vi "Read picture.vi"(8 "error in (no error)":errorcluster, 11 "data_loader in":refnum<class "data_loader.lvclass">) -> (0 "error out":errorcluster, 2 "picture":picture, 3 "data_loader out":refnum<class "data_loader.lvclass">)   [LabVIEW 2017, in "data_loader.lvclass"]
uses:
  data_loader.lvclass
  data_loader.lvclass/data_loader.ctl
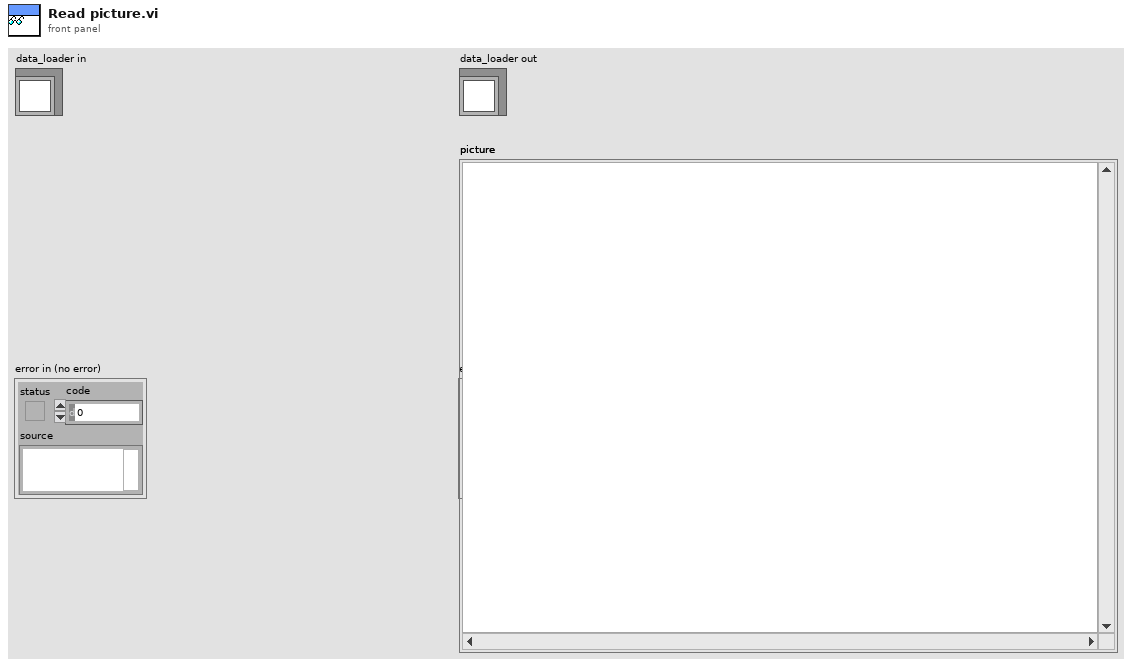
[diagram p1: front panel]
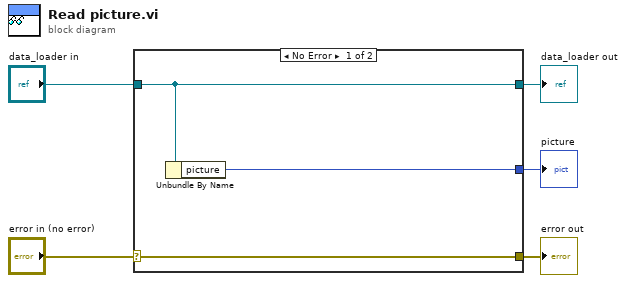
[diagram p0: block diagram]
diagram:
  n1 = case shown="No Error" "error in (no error)" {
    selector: "error in (no error)" -> [w8 w9]
    tunnel: [w8 w9] -> w4
    tunnel: [w7 w10] -> w2
    tunnel: "data_loader in" -> [w7 w10]
    tunnel: [w6 _] -> w1
    frame No Error {
      n2 = Unbundle By Name(w7) -> ("picture"=w6:picture)
    }
    frame Error {
    }
  }
  "error out" <- w4
  "data_loader out" <- w2
  "picture" <- w1
